vi "Banana_Disconnect TypeDef.vi"(6 "Skip type-def verification":bool, 8 "Variant":variant) -> (2 "Variant Out":variant)   [LabVIEW 2021, in "Bananas.lvlib"]
uses:
  Bananas.lvlib
  <vilib>/Utility/Data Type/NI_Data Type.lvlib
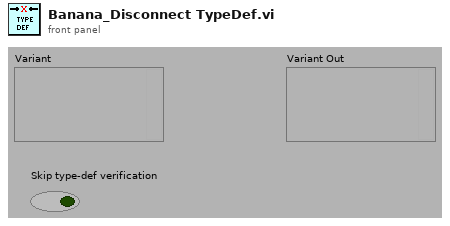
[diagram p1: front panel]
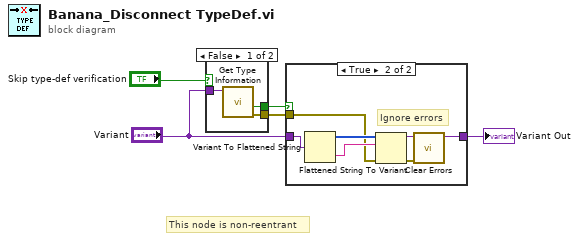
[diagram p0: block diagram]
diagram:
  # "This node is non-reentrant"
  n1 = case shown="False" "Skip type-def verification" {
    selector: "Skip type-def verification" -> [_ w9]
    tunnel: "Variant" -> [w8 _]
    tunnel: [w7 w9] -> w3
    tunnel: [w6 _] -> w2
    frame False {
      n2 = call <vilib>:"Get Type Information.vi"("variant"=w8) -> ("error out"=w6:errorcluster, "type definition"=w7:bool)  [unwired: 6 in, 3 out]
    }
    frame True {
    }
  }
  n3 = case shown="True" w3 {
    tunnel: [w10 w15] -> w5
    tunnel: "Variant" -> [w10 w12]
    tunnel: w2 -> [_ w11]
    frame False {
    }
    frame True {
      # "Ignore errors"
      n4 = Variant To Flattened String(Variant=w12) -> (data string=w13:string, 1:w14:i16[])
      n5 = Flattened String To Variant(4:w11, 6:w13, 7:w14) -> (0:w16:errorcluster, 3:w15:variant)
      n6 = call <vilib>:"Clear Errors.vi"("error in (no error)"=w16) -> ()  [unwired: 5 in, 2 out]
    }
  }
  "Variant Out" <- w5
